vi "KEI_Current.vi"(3 "error in":errorcluster, 4 "Language":T1, 5 "currentLsit":string="221", 6 "GPIB In":refnum<visa-resource-name>="GPIB0::16::INSTR") -> (0 "error out":errorcluster, 1 "Message":string, 2 "current":dbl)   [LabVIEW 2015]
uses:
  CustomControl/Lang_Control.ctl
  <instrlib>/Keithley 27XX/Public/Data/Read Single Point.vi
  <instrlib>/Keithley 27XX/Keithley 27XX.lvlib
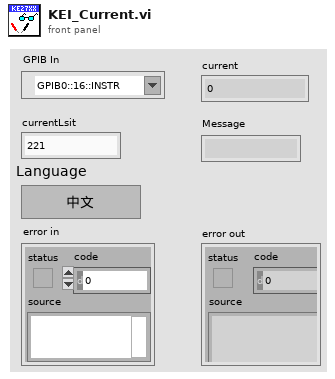
[diagram p1: front panel]
types:
  T1 = typedef "Lang_Control.ctl" = enum16{"中文", "English"}
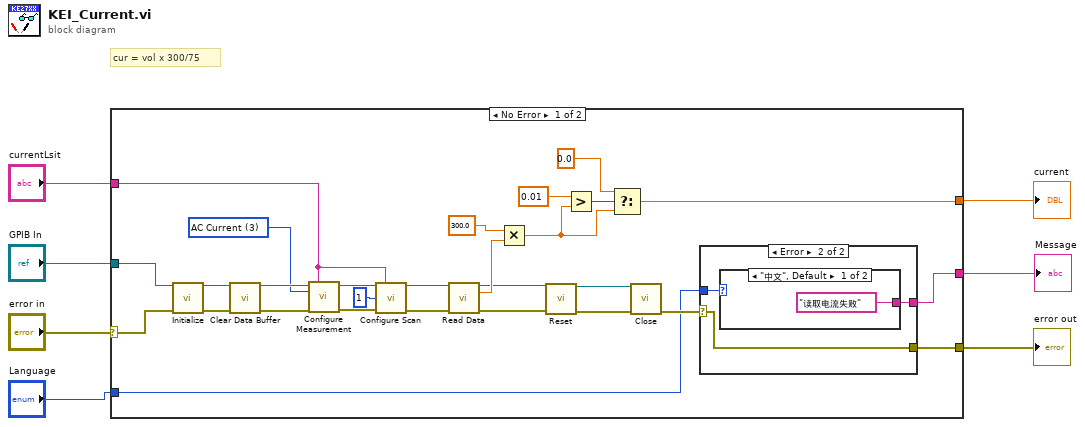
[diagram p0: block diagram]
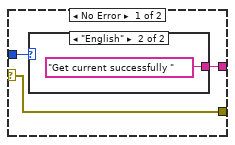
[diagram p2: hidden frame]
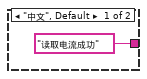
[diagram p3: hidden frame]
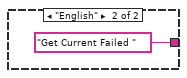
[diagram p4: hidden frame]
diagram:
  # "cur = vol x 300/75"
  n1 = case shown="No Error" "error in" {
    selector: "error in" -> [w17 w46]
    tunnel: "currentLsit" -> [w27 _]
    tunnel: "GPIB In" -> [w23 _]
    tunnel: [w19 _] -> w5
    tunnel: [w15 w46] -> w3
    tunnel: [w14 _] -> w2
    tunnel: "Language" -> [w13 _]
    frame No Error {
      w33 = u16 3 items=["DC Voltage", "AC Voltage", "DC Current", "AC Current", "Resistance", "Four-Wire Resistance", "Temperature", "Frequency", "Period", "Continuity"] ("Function (0: DC Voltage)")
      n2 = call <instrlib>:"Initialize.vi"("VISA resource name"=w23, "error in (no error)"=w17) -> ("VISA resource name out"=w25:refnum<visa-resource-name>, "error out"=w24:errorcluster)  [unwired: 12 in]
      n3 = call <instrlib>:"Clear Data Buffer.vi"("VISA resource name"=w25, "error in (no error)"=w24) -> ("VISA resource name out"=w35:refnum<visa-resource-name>, "error out"=w34:errorcluster)  [unwired: 12 in]
      n4 = call <instrlib>:"Configure Measurement.vi"("VISA resource name"=w35, "Scan List (Empty)"=w27, "Function (0: DC Voltage)"=w33, "error in (no error)"=w34) -> ("VISA resource name out"=w32:refnum<visa-resource-name>, "error out"=w31:errorcluster)  [unwired: 10 in]
      n5 = call <instrlib>:"Configure Scan.vi"("VISA resource name"=w32, "Channel List (101:110)"=w27, "Sample Count (100)"=1, "error in (no error)"=w31) -> ("VISA resource name out"=w29:refnum<visa-resource-name>, "error out"=w28:errorcluster)  [unwired: 10 in]
      n6 = call-poly <instrlib>:"Read Data.vi"("VISA resource name"=w29, "error in (no error)"=w28) -> ("VISA resource name out"=w9:refnum<visa-resource-name>, "Measurement Data"=w26:dbl, "error out"=w8:errorcluster)  [unwired: 11 in]
      n7 = Multiply(x=300.0, y=w26) -> (x*y=w12:dbl)
      n8 = call <instrlib>:"Reset.vi"("VISA resource name"=w9, "error in (no error)"=w8) -> ("VISA resource name out"=w11:refnum<visa-resource-name>, "error out"=w10:errorcluster)  [unwired: 12 in]
      n9 = Greater?(x=0.01 ("y"), y=w12) -> (0:w21:bool)
      n10 = Select(t=0.0, s=w21, f=w12) -> (s? t:f=w19:dbl)
      n11 = call <instrlib>:"Close.vi"("VISA resource name"=w11, "error in (no error)"=w10) -> ("error out"=w16:errorcluster)  [unwired: 13 in]
      n12 = case shown="Error" w16 {
        selector: w16 -> [w37 w42]
        tunnel: [w38 w43] -> w14
        tunnel: [w37 w42] -> w15
        tunnel: w13 -> [w36 w41]
        frame No Error {
          n13 = case shown="\"English\"" w36 {
            tunnel: ["读取电流成功" "Get current successfully "] -> w38
            frame "中文", Default {
            }
            frame "English" {
            }
          }
        }
        frame Error {
          n14 = case shown="\"中文\", Default" w41 {
            tunnel: ["读取电流失败" "Get Current Failed "] -> w43
            frame "中文", Default {
            }
            frame "English" {
            }
          }
        }
      }
    }
    frame Error {
    }
  }
  "error out" <- w3
  "current" <- w5
  "Message" <- w2
